vi "Part 2.vi"(11 "Input":string) -> (3 "Output":i64)   [LabVIEW 2021]
uses:
  <userlib>/_OpenG.lib/array/array.llb/Search 1D Array (I64)__ogtk.vi
panel:
  out "Grid":i64[][](array[numeric])
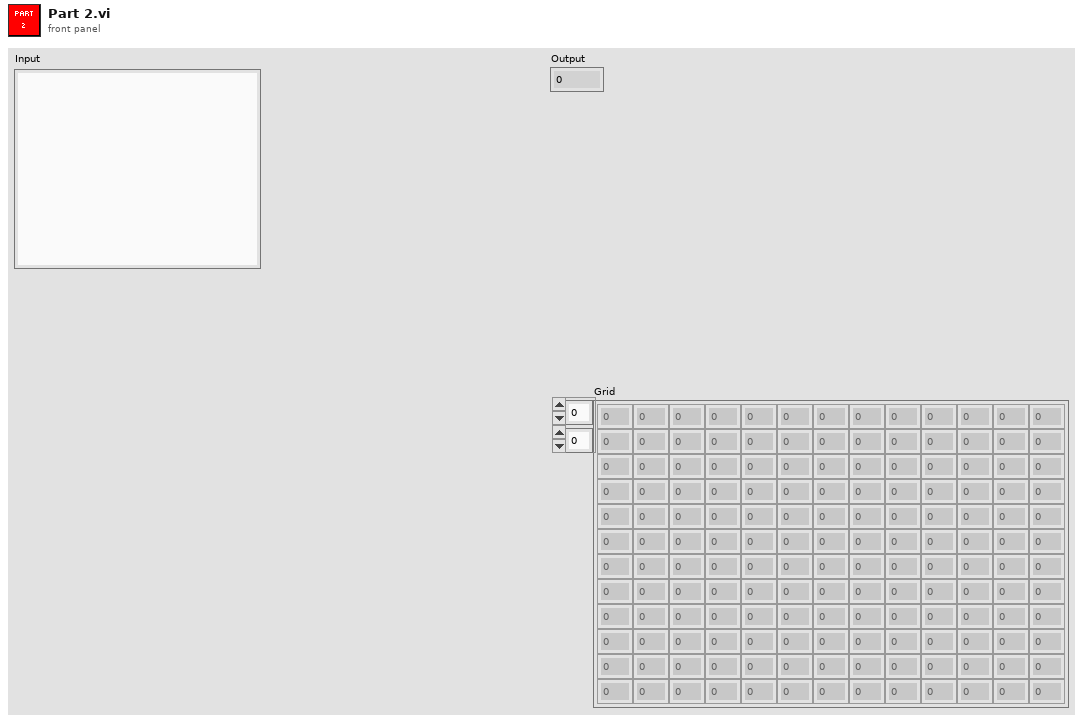
[diagram p1: front panel]
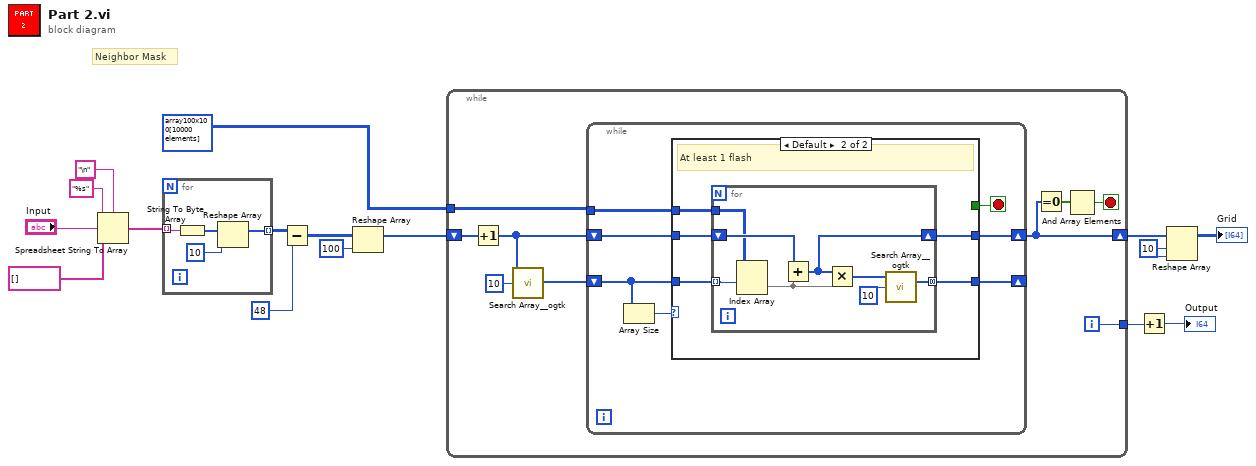
[diagram p0: block diagram]
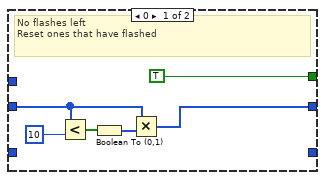
[diagram p2: hidden frame]
diagram:
  w4 = 10 ("dimension size")
  # "Neighbor Mask"
  n1 = Spreadsheet String To Array(delimiter (Tab)="\n", format string="%s", spreadsheet string="Input", array type (2D Dbl)=string[] []) -> (array=w12:string[])
  n2 = for {
    tunnel: w12 -> [w20] mode=indexing
    tunnel: [w18] -> w11 mode=indexing
    n3 = String To Byte Array(string=w20) -> (unsigned byte array=w19:u8[])
    n4 = Reshape Array(w19, 10 ("dimension size")) -> (w18:u8[])
  }
  n5 = Subtract(x=w11, y=i64 48) -> (x-y=w9:i64[][])
  n6 = Reshape Array(w9, 100 ("dimension size")) -> (w7:i64[])
  n7 = while {
    shift-right: [w22] -> w8
    shift-left: w7 -> [w29]
    tunnel: i16[][] array100x100[10000 elements] ("Array") -> [w25]
    tunnel: [w24] -> w2
    i -> [w24]
    stop <- w21 stop-if-true
    n8 = Increment(x=w29) -> (x+1=w28:i64[])
    n9 = call-poly <userlib>:"Search Array__ogtk.vi"("Array"=w28, "Element Data"=i64 10) -> ("Indices of Elements"=w26:i32[])  [unwired: 7 in]
    n10 = while {
      shift-right: [w36] -> w22
      shift-left: w28 -> [w33]
      shift-right: [w32] -> _
      shift-left: w26 -> [w34]
      tunnel: w25 -> [w30]
      stop <- w35 stop-if-true
      n11 = Array Size(array=w34) -> (size(s)=w31:i32)
      n12 = case shown="Default" w31 {
        tunnel: [w37 w45] -> w36
        tunnel: [TRUE _] -> w35
        tunnel: w34 -> [_ w47]
        tunnel: w33 -> [w38 w46]
        tunnel: [_ w44] -> w32
        tunnel: w30 -> [_ w43]
        frame 0 {
          # "No flashes left\nReset ones that have flashed"
          n13 = Less?(x=w38, y=i64 10) -> (x < y?=w41:bool[])
          n14 = Boolean To (0,1)(Boolean=w41) -> (0, 1=w40:i16[])
          n15 = Multiply(x=w38, y=w40) -> (x*y=w37:i64[])
        }
        frame Default {
          # "At least 1 flash"
          n16 = for {
            tunnel: w47 -> [w53] mode=indexing
            shift-right: [w51] -> w45
            shift-left: w46 -> [w52]
            tunnel: [w55] -> w44 mode=concatenating
            tunnel: w43 -> [w50]
            n17 = Index Array(array=w50, index (row)=w53) -> (element=w49:i16[])  [unwired: 1 in]
            n18 = Add(x=w52, y=w49) -> (x+y=w51:i64[])
            n19 = Multiply(x=w51, y=w49) -> (x*y=w48:i64[])
            n20 = call-poly <userlib>:"Search Array__ogtk.vi"("Array"=w48, "Element Data"=i64 10) -> ("Indices of Elements"=w55:i32[])  [unwired: 7 in]
          }
        }
      }
    }
    n21 = Equal To 0?(x=w22) -> (x = 0?=w23:bool[])
    n22 = And Array Elements(Boolean array=w23) -> (logical AND=w21:bool)
  }
  n23 = Increment(x=w2) -> (x+1=→"Output":i32)
  n24 = Reshape Array(w8, w4, w4) -> (→"Grid":i64[][])
